vi "Initialize.vi"(6 "Start Direction":T1=enum."E", 8 "error in (no error)":errorcluster, 9 "Kamikaze DVR":T2, 10 "SquareStatus DVR":T3, 11 "Mother in":refnum<class "Mother.lvclass">) -> (0 "error out":errorcluster, 3 "Mother out":refnum<class "Mother.lvclass">)   [LabVIEW 2014, in "Mother.lvclass"]
uses:
  Mother.lvclass
  SquareStatus DVR.ctl
  Kamikaze DVR.ctl
  Direction Enum.ctl
  Mother.lvclass/Mother.ctl
  SquareBattle.lvclass
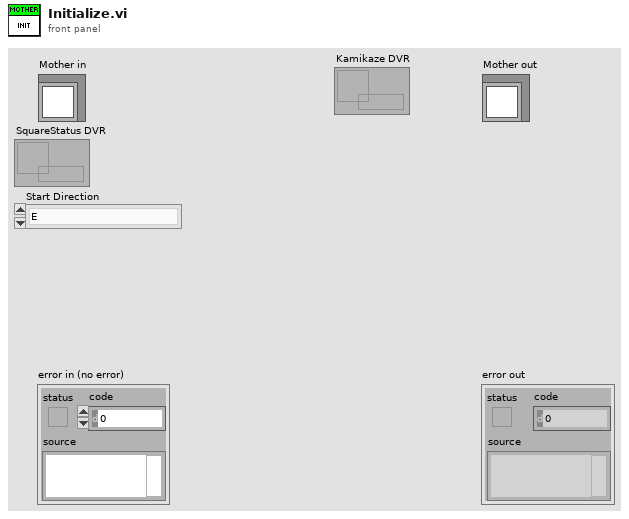
[diagram p1: front panel]
types:
  T1 = typedef "SquareBattle.lvclass/Direction Enum.ctl" = enum16{"NW", "N", "NE", "E", "SE", "S", "SW", "W"}
  T2 = typedef "Kamikaze DVR.ctl" = refnum<data-value>
  T3 = typedef "Mother.lvclass/SquareStatus DVR.ctl" = refnum<data-value>
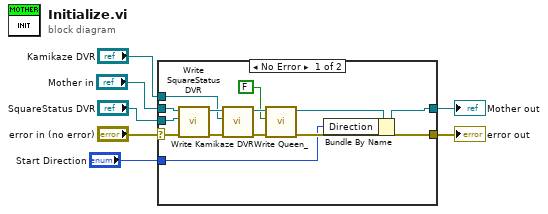
[diagram p0: block diagram]
diagram:
  n1 = case shown="No Error" "error in (no error)" {
    selector: "error in (no error)" -> [w20 w22]
    tunnel: [w13 w22] -> w6
    tunnel: [w9 w21] -> w4
    tunnel: "Mother in" -> [w18 w21]
    tunnel: "SquareStatus DVR" -> [w17 _]
    tunnel: "Kamikaze DVR" -> [w14 _]
    tunnel: "Start Direction" -> [w8 _]
    frame No Error {
      n2 = call-dynamic "Write SquareStatus DVR.vi"("error in (no error)"=w20, "data value reference"=w17, "Mother in"=w18) -> ("error out"=w19:errorcluster, "Mother out"=w15:refnum<class "Mother.lvclass">)  [unwired: 7 in]
      n3 = call "Write Kamikaze DVR.vi"("error in (no error)"=w19, "Kamikaze DVR"=w14, "Mother in"=w15) -> ("error out"=w16:errorcluster, "Mother out"=w12:refnum<class "Mother.lvclass">)  [unwired: 7 in]
      n4 = call "Write Queen_.vi"("error in (no error)"=w16, "Queen?"=FALSE, "Mother in"=w12) -> ("error out"=w13:errorcluster, "Mother out"=w11:refnum<class "Mother.lvclass">)  [unwired: 7 in]
      n5 = Bundle By Name(cluster=w11, "Direction"=w8) -> (w9:refnum<class "Mother.lvclass">)
    }
    frame Error {
    }
  }
  "error out" <- w6
  "Mother out" <- w4
